vi "RandomArray.vi"(1 "random array size":i32=256, 2 "factor":dbl=1.0) -> (0 "random array":dbl[](array[numeric]))   [LabVIEW 2014, in "examples.lvlib"]
uses:
  examples.lvlib
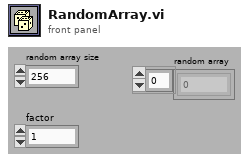
[diagram p1: front panel]
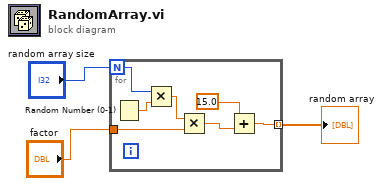
[diagram p0: block diagram]
diagram:
  n1 = for {
    N: "random array size" -> [w9]
    tunnel: "factor" -> [w8]
    tunnel: [w4] -> w1 mode=indexing
    n2 = Random Number (0-1)() -> (number: 0 to 1=w10:dbl)
    n3 = Multiply(x=w9, y=w10) -> (x*y=w7:dbl)
    n4 = Multiply(x=w7, y=w8) -> (x*y=w6:dbl)
    n5 = Add(x=15.0, y=w6) -> (x+y=w4:dbl)
  }
  "random array" <- w1
